vi "WriteIOValues gas.vi"(2 "error in":errorcluster, 3 "Output - Cluster gas":T1 {"GM TS-2[°C]" format="%.2g"; "GM TS-1 [°C]" format="%.4g"; "GM DS-1 [bar]" format="%.4g"; "GM DS-2 [bar]" format="%.2g"; "GM GZ-1 [imp]" format="%.2g"}, 5 "input cluster":T2) -> (0 "error out":errorcluster, 1 "Output - Cluster gas 2":T1 {"GM TS-2[°C]" format="%.2g"; "GM TS-1 [°C]" format="%.4g"; "GM DS-1 [bar]" format="%.4g"; "GM DS-2 [bar]" format="%.2g"; "GM GZ-1 [imp]" format="%.2g"})   [LabVIEW 2011]
uses:
  Input - Cluster gas.ctl
  Output - Cluster gas.ctl
panel:
  # "converted bool array!"
  # "mode :\n0: nothing\n1: quality\n2: quantity\n3: quality and quantity"
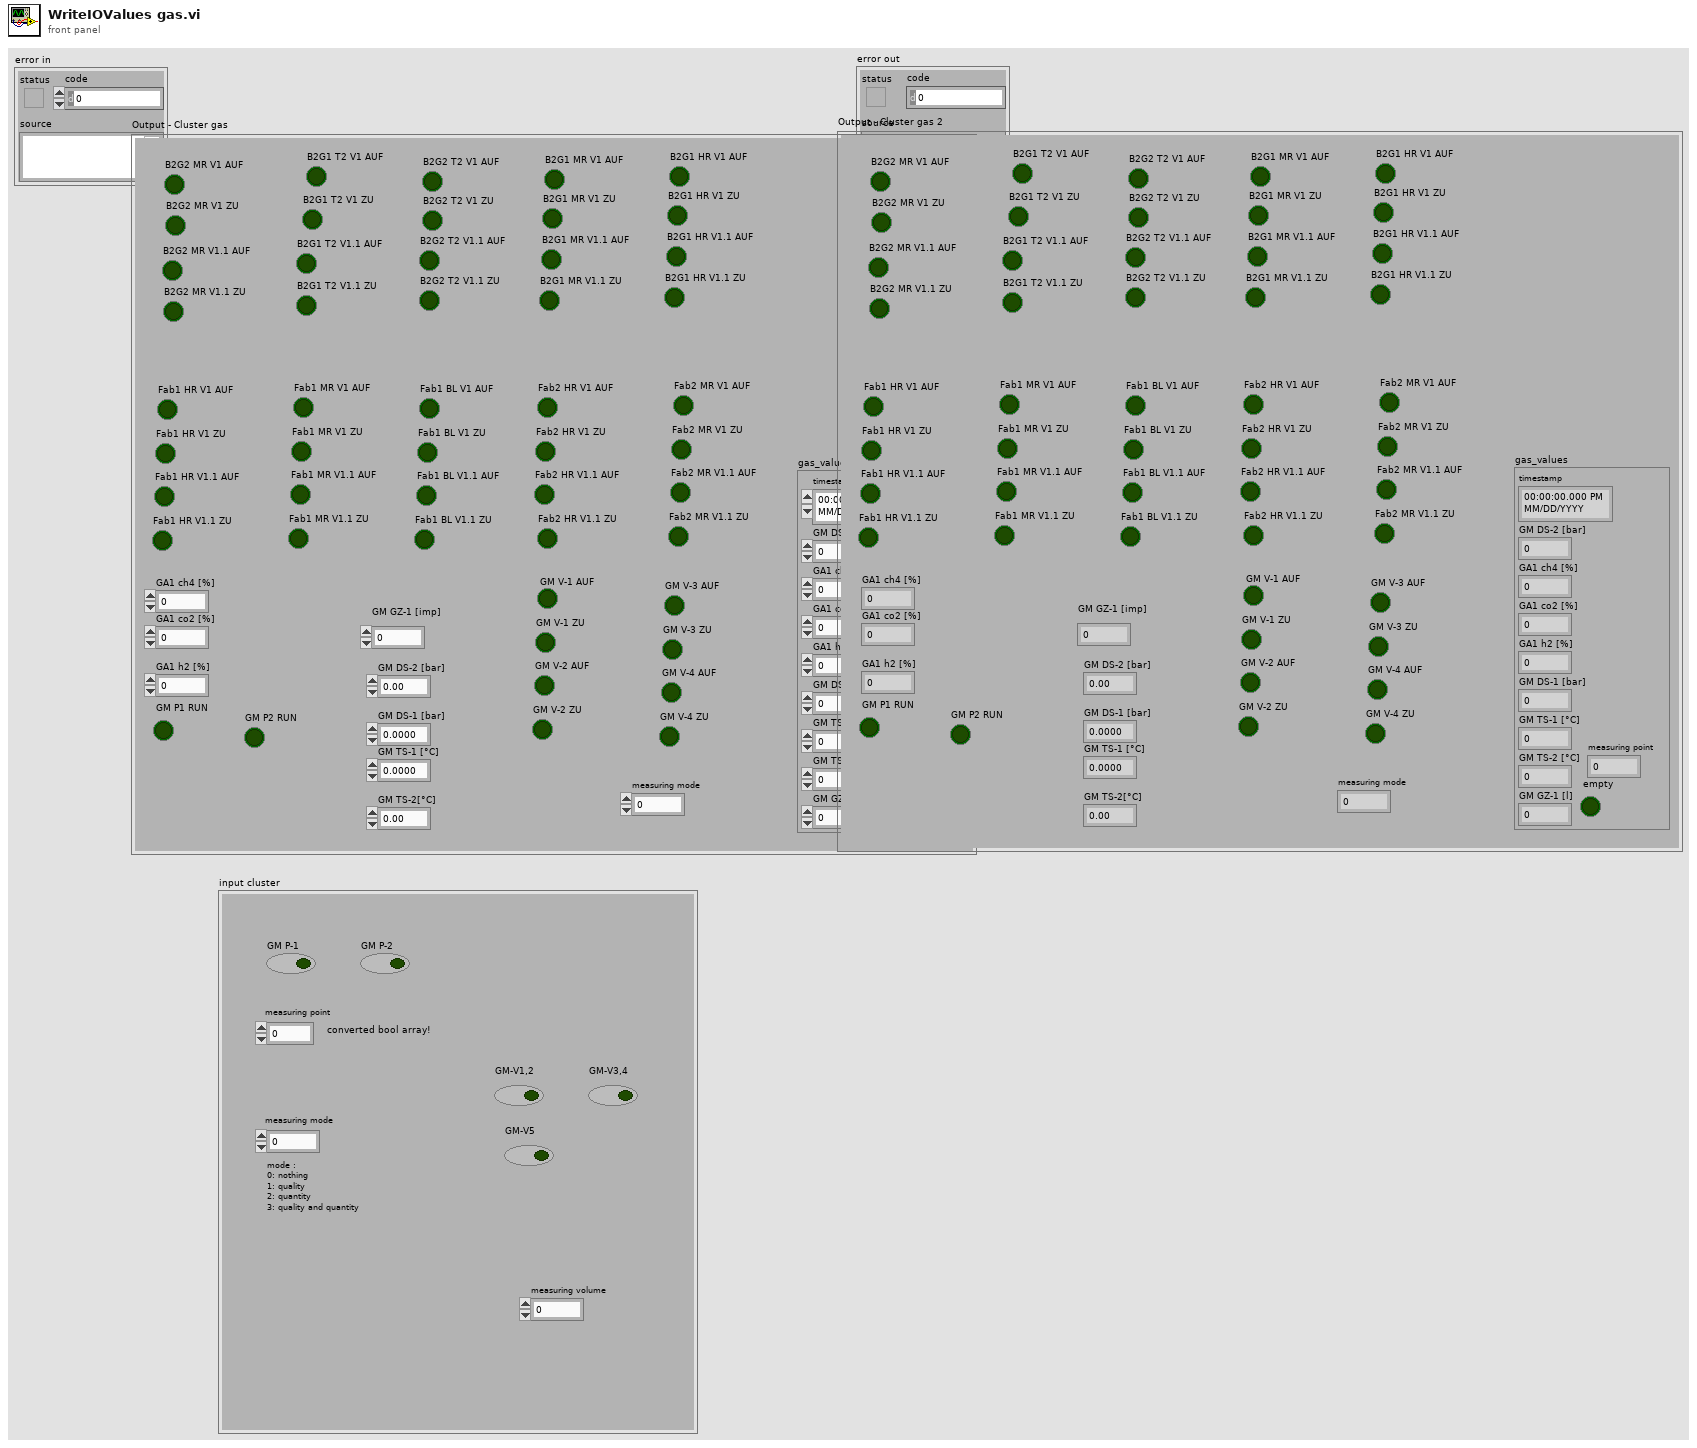
[diagram p1: front panel]
types:
  T1 = typedef "Output - Cluster gas.ctl" = cluster{"B2G2 MR V1.1 AUF":bool, "B2G2 MR V1.1 ZU":bool, "B2G2 MR V1 AUF":bool, "B2G2 MR V1 ZU":bool, "B2G1 T2 V1 AUF":bool, "B2G1 T2 V1 ZU":bool, "B2G1 T2 V1.1 AUF":bool, "B2G1 T2 V1.1 ZU":bool, "B2G2 T2 V1 AUF":bool, "B2G2 T2 V1 ZU":bool, "B2G2 T2 V1.1 ZU":bool, "B2G2 T2 V1.1 AUF":bool, "B2G1 MR V1 AUF":bool, "B2G1 MR V1 ZU":bool, "B2G1 MR V1.1 AUF":bool, "B2G1 MR V1.1 ZU":bool, "B2G1 HR V1 AUF":bool, "B2G1 HR V1 ZU":bool, "B2G1 HR V1.1 AUF":bool, "B2G1 HR V1.1 ZU":bool, "Fab1 HR V1 AUF":bool, "Fab1 HR V1 ZU":bool, "Fab1 HR V1.1 AUF":bool, "Fab1 HR V1.1 ZU":bool, "Fab1 MR V1 AUF":bool, "Fab1 MR V1 ZU":bool, "Fab1 MR V1.1 AUF":bool, "Fab1 MR V1.1 ZU":bool, "Fab1 BL V1 AUF":bool, "Fab1 BL V1 ZU":bool, "Fab1 BL V1.1 AUF":bool, "Fab1 BL V1.1 ZU":bool, "Fab2 HR V1 AUF":bool, "Fab2 HR V1 ZU":bool, "Fab2 HR V1.1 AUF":bool, "Fab2 HR V1.1 ZU":bool, "Fab2 MR V1 AUF":bool, "Fab2 MR V1 ZU":bool, "Fab2 MR V1.1 AUF":bool, "Fab2 MR V1.1 ZU":bool, "GA1 ch4 [%]":dbl, "GA1 co2 [%]":dbl, "GA1 h2 [%]":dbl, "GM P1 RUN":bool, "GM V-1 AUF":bool, "GM V-1 ZU":bool, "GM V-2 AUF":bool, "GM V-2 ZU":bool, "GM V-3 AUF":bool, "GM V-3 ZU":bool, "GM V-4 AUF":bool, "GM V-4 ZU":bool, "GM P2 RUN":bool, "GM GZ-1 [imp]":u32, "GM DS-2 [bar]":dbl, "GM DS-1 [bar]":dbl, "GM TS-1 [°C]":dbl, "GM TS-2[°C]":dbl, "gas_values":cluster{"timestamp":timestamp, "GM DS-2 [bar]":dbl, "GA1 ch4 [%]":dbl, "GA1 co2 [%]":dbl, "GA1 h2 [%]":dbl, "GM DS-1 [bar]":dbl, "GM TS-1 [°C]":dbl, "GM TS-2 [°C]":dbl, "GM GZ-1 [l]":dbl, "empty":bool, "measuring point":u8}, "measuring mode":u8}
  T2 = typedef "Input - Cluster gas.ctl" = cluster{"GM P-1":bool, "GM P-2":bool, "measuring point":u32, "measuring mode":u8, "GM-V1,2":bool, "GM-V3,4":bool, "GM-V5":bool, "measuring volume":u32}
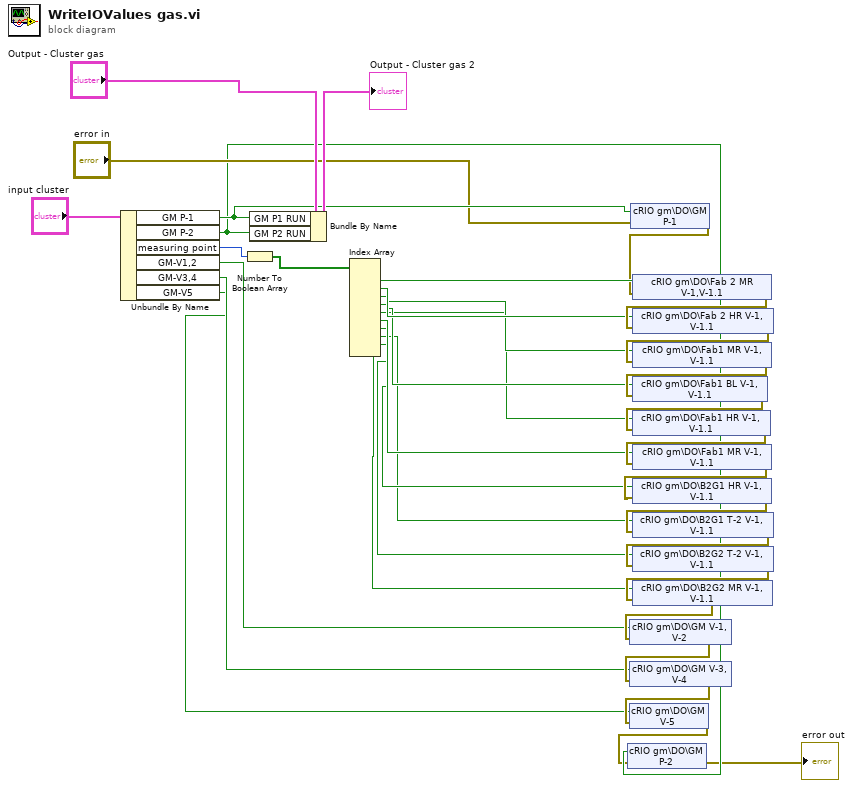
[diagram p0: block diagram]
diagram:
  n1 = Unbundle By Name("input cluster") -> ("GM P-1"=w12:bool, "GM P-2"=w4:bool, "measuring point"=w33:u32, "GM-V1,2"=w6:bool, "GM-V3,4"=w5:bool, "GM-V5"=w1:bool)
  n2 = Number To Boolean Array(number=w33) -> (Boolean array=w32:bool[])
  n3 = Bundle By Name(cluster="Output - Cluster gas", "GM P1 RUN"=w12, "GM P2 RUN"=w4) -> (→"Output - Cluster gas 2":T1)
  n4 = Index Array(array=w32) -> (element #1=w22:bool, element #2=w21:bool, element #3=w20:bool, element #4=w19:bool, element #5=w18:bool, element #6=w17:bool, element #7=w16:bool, element #8=w15:bool, element #9=w14:bool, element #10=w13:bool)  [unwired: 10 in]
  n5 = shared-variable "cRIO gm\\DO\\GM P-1"(w12, error in="error in") -> (error out=w11:errorcluster)
  n6 = shared-variable "cRIO gm\\DO\\Fab 2 MR V-1,V-1.1"(w22, error in=w11) -> (error out=w31:errorcluster)
  n7 = shared-variable "cRIO gm\\DO\\Fab 2 HR V-1, V-1.1"(w21, error in=w31) -> (error out=w30:errorcluster)
  n8 = shared-variable "cRIO gm\\DO\\Fab1 MR V-1, V-1.1"(w20, error in=w30) -> (error out=w29:errorcluster)
  n9 = shared-variable "cRIO gm\\DO\\Fab1 BL V-1, V-1.1"(w19, error in=w29) -> (error out=w28:errorcluster)
  n10 = shared-variable "cRIO gm\\DO\\Fab1 HR V-1, V-1.1"(w18, error in=w28) -> (error out=w27:errorcluster)
  n11 = shared-variable "cRIO gm\\DO\\Fab1 MR V-1, V-1.1"(w17, error in=w27) -> (error out=w26:errorcluster)
  n12 = shared-variable "cRIO gm\\DO\\B2G1 HR V-1, V-1.1"(w16, error in=w26) -> (error out=w25:errorcluster)
  n13 = shared-variable "cRIO gm\\DO\\B2G1 T-2 V-1, V-1.1"(w15, error in=w25) -> (error out=w24:errorcluster)
  n14 = shared-variable "cRIO gm\\DO\\B2G2 T-2 V-1, V-1.1"(w14, error in=w24) -> (error out=w23:errorcluster)
  n15 = shared-variable "cRIO gm\\DO\\B2G2 MR V-1, V-1.1"(w13, error in=w23) -> (error out=w9:errorcluster)
  n16 = shared-variable "cRIO gm\\DO\\GM V-1, V-2"(w6, error in=w9) -> (error out=w8:errorcluster)
  n17 = shared-variable "cRIO gm\\DO\\GM V-3, V-4"(w5, error in=w8) -> (error out=w7:errorcluster)
  n18 = shared-variable "cRIO gm\\DO\\GM V-5"(w1, error in=w7) -> (error out=w2:errorcluster)
  n19 = shared-variable "cRIO gm\\DO\\GM P-2"(w4, error in=w2) -> (error out=→"error out":errorcluster)
